vi "Read Gantry.vi"(8 "error in (no error)":errorcluster, 11 "Tool Class in":refnum<class "Tool Class.lvclass">) -> (0 "error out":errorcluster, 2 "Gantry Class.lvclass":refnum<class "Gantry Class.lvclass">, 3 "Tool Class out":refnum<class "Tool Class.lvclass">)   [LabVIEW 2011, in "Tool Class.lvclass"]
uses:
  Tool Class.lvclass
  Gantry Class/Gantry Class.lvclass
  Tool Class.lvclass/Tool Class.ctl
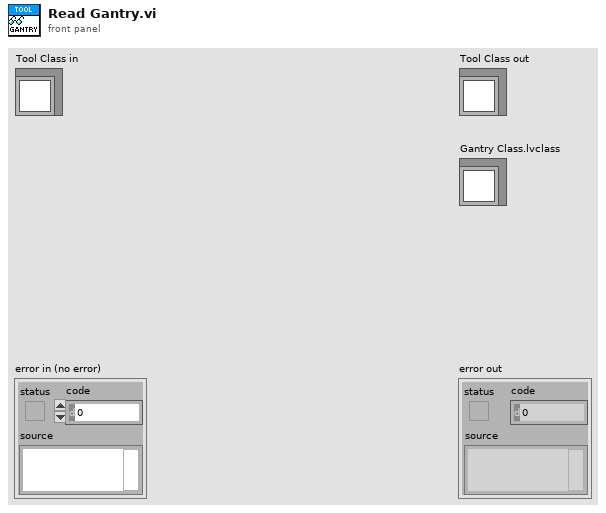
[diagram p1: front panel]
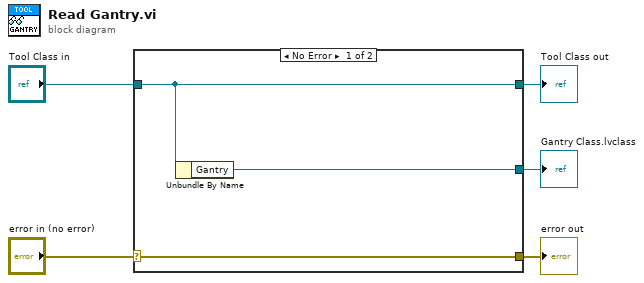
[diagram p0: block diagram]
diagram:
  n1 = case shown="No Error" "error in (no error)" {
    selector: "error in (no error)" -> [w8 w9]
    tunnel: [w8 w9] -> w4
    tunnel: [w7 w10] -> w2
    tunnel: "Tool Class in" -> [w7 w10]
    tunnel: [w6 _] -> w1
    frame No Error {
      n2 = Unbundle By Name(w7) -> ("Gantry"=w6:refnum<class "Gantry Class.lvclass">)
    }
    frame Error {
    }
  }
  "error out" <- w4
  "Tool Class out" <- w2
  "Gantry Class.lvclass" <- w1
